vi "Log VNA Data - TDMS.vi"(4 "error in (no error)":errorcluster, 7 "Data in":T1 {"LogStartTime" format="%<%x %.3X>T"}) -> (0 "error out":errorcluster, 3 "Data out":T1 {"LogStartTime" format="%<%x %.3X>T"})   [LabVIEW 2023]
uses:
  controls/UI Data.ctl
  <vilib>/NI/Modbus Library/API/Master/Modbus Master.lvclass
  LibreVNA/LibreVNA.lvclass
panel:
  out "resulting string":string
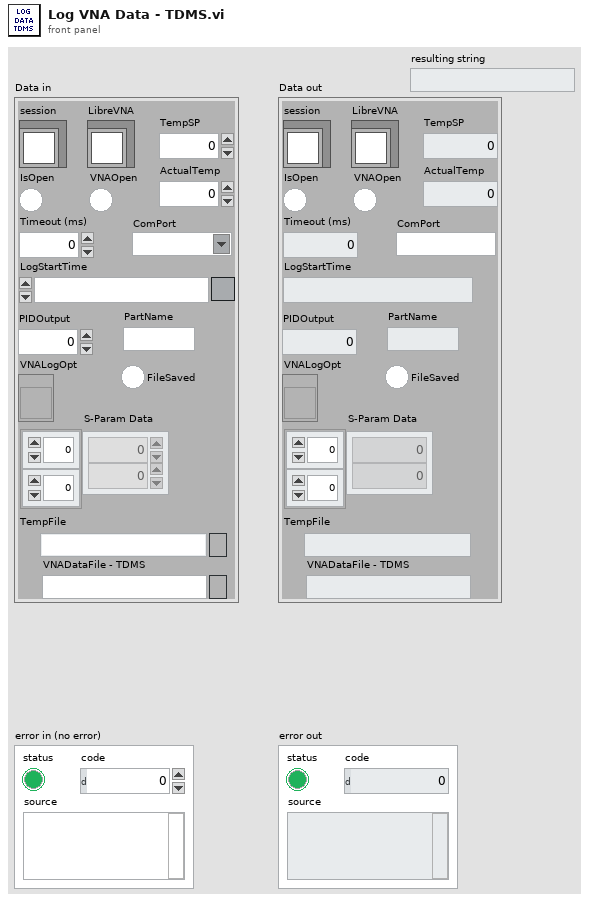
[diagram p1: front panel]
types:
  T1 = typedef "UI Data.ctl" = cluster{"session":refnum<class "Modbus Master.lvclass">, "IsOpen":bool, "Timeout (ms)":i32, "TempFile":path, "LogStartTime":timestamp, "LibreVNA":refnum<class "LibreVNA.lvclass">, "VNAOpen":bool, "TempSP":dbl, "ActualTemp":dbl, "FileSaved":bool, "PIDOutput":dbl, "VNALogOpt":refnum<vi>, "PartName":string, "ComPort":refnum<visa-resource-name>, "S-Param Data":dbl[][], "VNADataFile - TDMS":path}
  T2 = enum16{"open", "open or create", "create or replace", "create", "open (read-only)"}
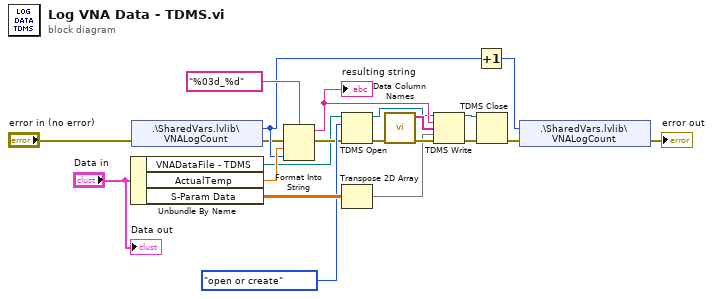
[diagram p0: block diagram]
diagram:
  n1 = Unbundle By Name("Data in") -> ("VNADataFile - TDMS"=w7:path, "ActualTemp"=w19:dbl, "S-Param Data"=w17:dbl[][])
  n2 = shared-variable ".\\SharedVars.lvlib\\VNALogCount"(error in="error in (no error)") -> (w6:u32, error out=w2:errorcluster)
  n3 = Format Into String(format string="%03d_%d", error in=w2, w19, w6) -> (resulting string=w11:string, error out=w12:errorcluster)  [unwired: 1 in]
  "resulting string" <- w11
  n4 = TDMS Open(8:w12, 10:T2."open or create" ("operation (0:open)"), 11:w7) -> (0:w21:errorcluster, 3:w9:refnum<k34>)  [unwired: 4 in]
  n5 = Transpose 2D Array(2D array=w17) -> (transposed array=w14:dbl[][])
  n6 = call "Data Column Names.vi"("error in"=w21) -> ("error out"=w15:errorcluster, "Array"=w16:string[])  [unwired: 5 in]
  n7 = TDMS Write(0:w9, 5:w11, 7:w16, 9:w14, 11:w15) -> (4:w10:refnum<k34>, 15:w8:errorcluster)  [unwired: 1 in, 2 out]
  n8 = Increment(x=w6) -> (x+1=w5:u32)
  n9 = TDMS Close(8:w8, 11:w10) -> (0:w4:errorcluster)  [unwired: 1 out]
  n10 = shared-variable ".\\SharedVars.lvlib\\VNALogCount"(w5, error in=w4) -> (error out=→"error out":errorcluster)
  "Data out" <- "Data in"
